vi "System Audit.vi"(3 "Sytem #":u8=1 min=1 max=16, 4 "AutoAge.ini  File Path":path=path "\\\\Beco\\autoage/config/autoage.ini", 5 "Status In":bool) -> (2 "Status Out":bool)   [LabVIEW 2021]
panel:
  out "time string":string
  out "date string":string
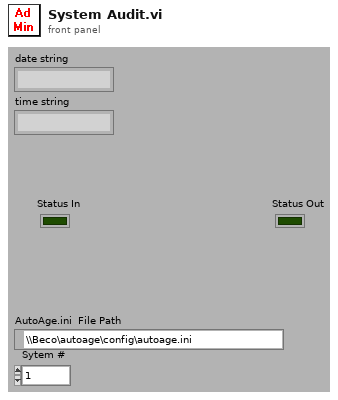
[diagram p1: front panel]
types:
  T1 = enum16{"open", "open or create", "create or replace", "create", "open (read only)"}
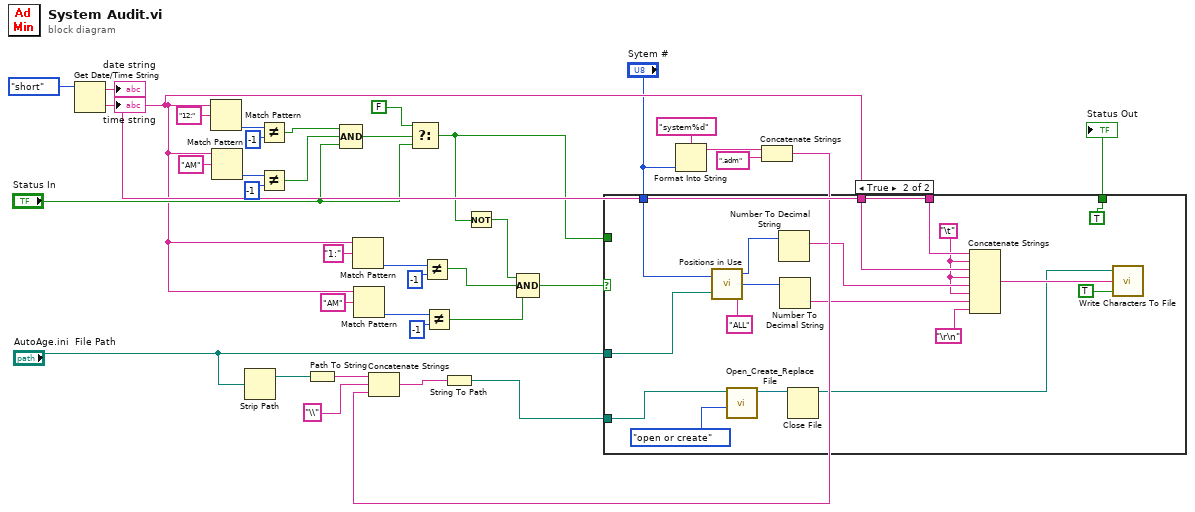
[diagram p0: block diagram]
diagram:
  n1 = Get Date/Time String(date format (0)=enum16{"short", "long", "abbreviated"}."short") -> (date string=w36:string, time string=w14:string)  [unwired: 2 in]
  "date string" <- w36
  "time string" <- w14
  n2 = Match Pattern(string=w14, regular expression="12:") -> (offset past match=w30:i32)  [unwired: 1 in, 3 out]
  n3 = Match Pattern(string=w14, regular expression="AM") -> (offset past match=w33:i32)  [unwired: 1 in, 3 out]
  n4 = Strip Path(path="AutoAge.ini  File Path") -> (stripped path=w12:path)  [unwired: 1 out]
  n5 = Not Equal?(x=w30, y=-1) -> (x != y?=w29:bool)
  n6 = Not Equal?(x=w33, y=-1) -> (x != y?=w28:bool)
  n7 = Path To String(path=w12) -> (string=w7:string)
  n8 = Compound Arithmetic op=AND(w29, w28, "Status In") -> (w27:bool)
  n9 = Match Pattern(string=w14, regular expression="1:") -> (offset past match=w22:i32)  [unwired: 1 in, 3 out]
  n10 = Match Pattern(string=w14, regular expression="AM") -> (offset past match=w20:i32)  [unwired: 1 in, 3 out]
  n11 = Select(t=FALSE, s=w27, f="Status In") -> (s? t:f=w2:bool)
  n12 = Not Equal?(x=w22, y=-1) -> (x != y?=w17:bool)
  n13 = Not Equal?(x=w20, y=-1) -> (x != y?=w18:bool)
  n14 = Not(x=w2) -> (.not. x?=w16:bool)
  n15 = Compound Arithmetic op=AND(w16, w17, w18) -> (w15:bool)
  n16 = Format Into String(format string="system%d" ("Format String"), "Sytem #") -> (resulting string=w9:string)  [unwired: 2 in, 1 out]
  n17 = Concatenate Strings(w9, ".adm" ("Substring")) -> (w4:string)
  n18 = Concatenate Strings(w7, "\\", w4) -> (w6:string)
  n19 = String To Path(string=w6) -> (path=w5:path)
  n20 = case shown="True" w15 {
    tunnel: "AutoAge.ini  File Path" -> [_ w53]
    tunnel: "Sytem #" -> [_ w52]
    tunnel: w36 -> [_ w51]
    tunnel: w14 -> [_ w50]
    tunnel: w5 -> [_ w43]
    tunnel: w2 -> [w38 _]
    tunnel: [w38 TRUE ("Status In")] -> w1
    frame False {
    }
    frame True {
      w46 = "\t"
      n21 = call "Positions in Use.vi"("Sytem #"=w52, "AutoAge.ini  File Path"=w53, "Oscillator Type"="ALL") -> ("Positions In Use"=w55:i32, "Total Positions"=w54:i32)
      n22 = call <vilib>:"Open_Create_Replace File.vi"("function (open:0)"=T1."open or create", "file path"=w43) -> ("refnum"=w41:refnum<file>)  [unwired: 6 in, 3 out]
      n23 = Number To Decimal String(number=w55) -> (decimal integer string=w49:string)  [unwired: 1 in]
      n24 = Number To Decimal String(number=w54) -> (decimal integer string=w48:string)  [unwired: 1 in]
      n25 = Close File(refnum=w41) -> (path=w40:path)  [unwired: 1 in, 1 out]
      n26 = Concatenate Strings(w51, w46, w50, w46, w49, w46, w48, "\r\n") -> (w45:string)
      n27 = call <vilib>:"Write Characters To File.vi"("append to file? (new file:F)"=TRUE, "character string"=w45, "file path (dialog if empty)"=w40) -> ()  [unwired: 2 in, 1 out]
    }
  }
  "Status Out" <- w1
